vi "Step Data Buffer.vi"(6 "config paths":T2, 7 "Mode":enum16{"Init", "Read", "Write"}(ring)=enum."Write", 8 "Error In":errorcluster, 9 "Step Hisitory In":string[](array[string]), 10 "Segment Data":T1, 11 "Add Step? In":bool) -> (0 "Error Out":errorcluster, 1 "Step Hisitory Out":string[](array[string]), 2 "Segment Data":T1, 3 "Add Step? Out":bool, 4 "config paths":T2)   [LabVIEW 2018]
uses:
  type defs/config paths for seq def.ctl
  type defs/Sequence Info.ctl
  type defs/Step Data Control.ctl
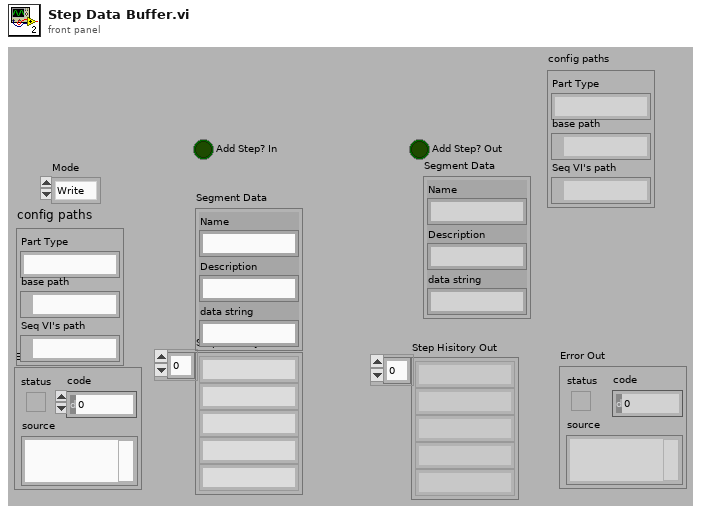
[diagram p1: front panel]
types:
  T1 = typedef "Sequence Info.ctl" = cluster{"Name":string, "Description":string, "data string":string}
  T2 = typedef "config paths for seq def.ctl" = cluster{"Part Type":string, "base path":path, "Seq VI's path":path}
  T3 = typedef "Step Data Control.ctl" = cluster{"Add Step?":bool, "Segment Data":T1, "Step Hisitory":string[], "Part Type":string, "base path":path}
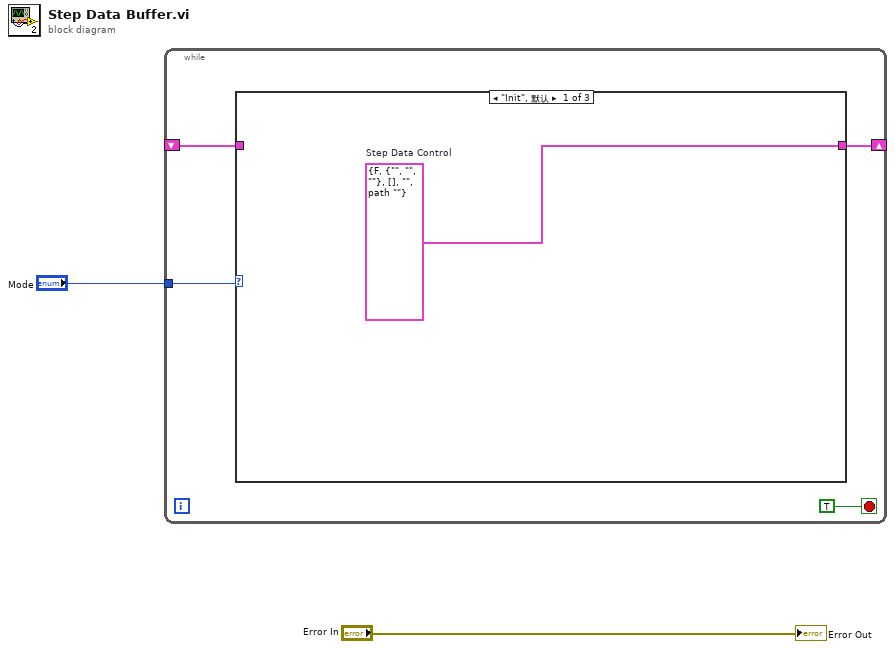
[diagram p0: block diagram]
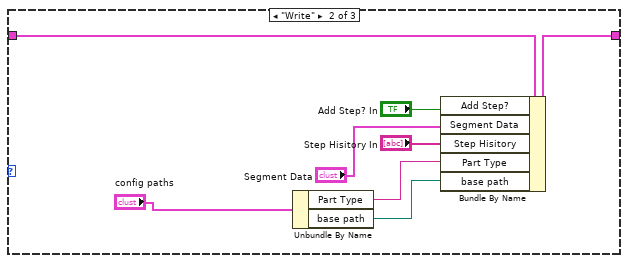
[diagram p2: hidden frame]
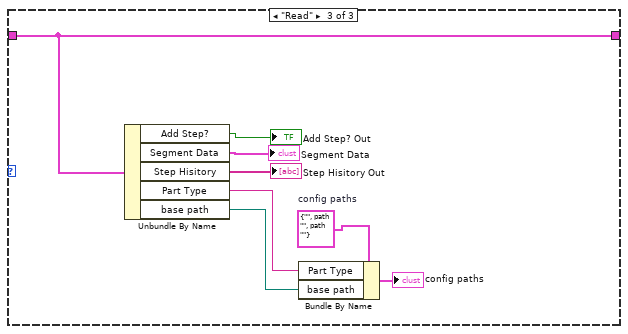
[diagram p3: hidden frame]
diagram:
  n1 = while {
    tunnel: "Mode" -> [w5]
    shift-right: [w4] -> _
    shift-left: _ -> [w3]
    stop <- TRUE stop-if-true
    n2 = case shown="\"Init\", 默认" w5 {
      tunnel: [w7 w14 w23] -> w4
      tunnel: w3 -> [_ w15 w23]
      frame "Init", Default {
        w7 = T3 {"Add Step?"=FALSE, "Segment Data"={"Name"="", "Description"="", "data string"=""}, "Step Hisitory"=[], "Part Type"="", "base path"=path ""}  # Step Data Control
      }
      frame "Write" {
        n3 = Unbundle By Name("config paths") -> ("Part Type"=w11:string, "base path"=w10:path)
        n4 = Bundle By Name(cluster=w15, "Add Step?"="Add Step? In", "Segment Data"="Segment Data", "Step Hisitory"="Step Hisitory In", "Part Type"=w11, "base path"=w10) -> (w14:T3)
      }
      frame "Read" {
        w16 = T2 {"Part Type"="", "base path"=path "", "Seq VI's path"=path ""}  # config paths
        n5 = Unbundle By Name(w23) -> ("Add Step?"=→"Add Step? Out":bool, "Segment Data"=→"Segment Data":T1, "Step Hisitory"=→"Step Hisitory Out":string[], "Part Type"=w19:string, "base path"=w18:path)
        n6 = Bundle By Name(cluster=w16, "Part Type"=w19, "base path"=w18) -> (→"config paths":T2)
      }
    }
  }
  "Error Out" <- "Error In"
